vi "APD_Order.vi"(2 "APD 4":bool, 3 "APD 3":bool, 4 "APD 2":bool, 5 "APD 1":bool) -> (0 "Detectors":i32[](array[numeric]), 1 "size(s)":i32)   [LabVIEW 2010]
doc: "From combination of activated switches, outputs number of active detectors (integer) and an array with all combinations of active detectors, the values of which are set to be correctly interpreted by the FPGA."
panel:
  # "This VI outputs the number of detectors (integer) and the array\ncorresponding to all combinations of active detectors, the values\nof which are set to be correctly interpreted by the FPGA."
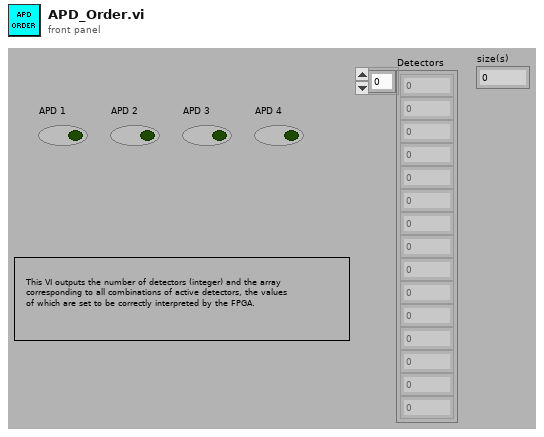
[diagram p1: front panel]
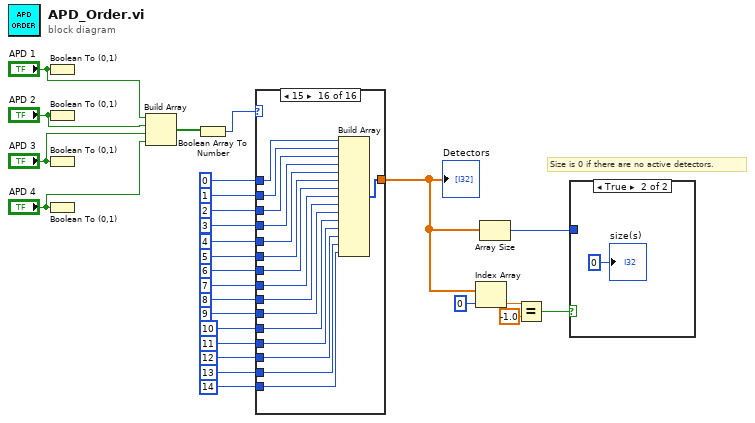
[diagram p0: block diagram]
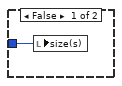
[diagram p2: hidden frame]
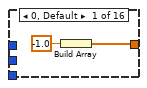
[diagram p3: hidden frame]
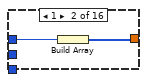
[diagram p4: hidden frame]
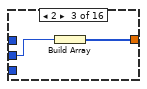
[diagram p5: hidden frame]
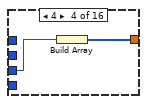
[diagram p6: hidden frame]
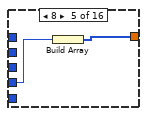
[diagram p7: hidden frame]
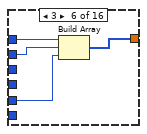
[diagram p8: hidden frame]
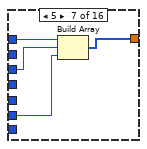
[diagram p9: hidden frame]
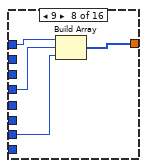
[diagram p10: hidden frame]
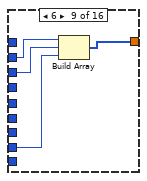
[diagram p11: hidden frame]
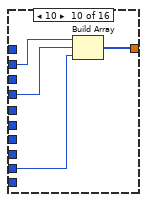
[diagram p12: hidden frame]
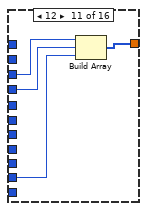
[diagram p13: hidden frame]
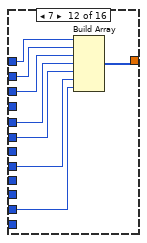
[diagram p14: hidden frame]
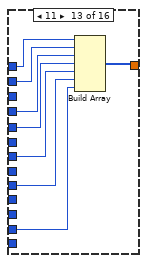
[diagram p15: hidden frame]
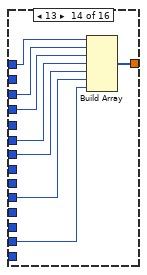
[diagram p16: hidden frame]
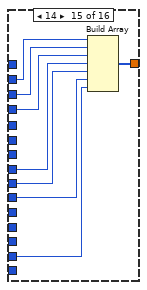
[diagram p17: hidden frame]
diagram:
  # "Size is 0 if there are no active detectors."
  n1 = Boolean To (0,1)(Boolean="APD 1") -> ()  [unwired: 1 out]
  n2 = Boolean To (0,1)(Boolean="APD 2") -> ()  [unwired: 1 out]
  n3 = Boolean To (0,1)(Boolean="APD 3") -> ()  [unwired: 1 out]
  n4 = Boolean To (0,1)(Boolean="APD 4") -> ()  [unwired: 1 out]
  n5 = Build Array("APD 1", "APD 2", "APD 3", "APD 4") -> (w26:bool[])
  n6 = Boolean Array To Number(Boolean array=w26) -> (number=w22:u32)
  n7 = case shown="15" w22 {
    tunnel: 0 -> [_ w31 _ _ _ w41 w45 w48 _ _ _ w69 w77 w85 _ w109]
    tunnel: 1 -> [_ _ w33 _ _ w40 _ _ w53 w57 _ w68 w75 _ w93 w108]
    tunnel: 2 -> [_ _ _ w35 _ _ w43 _ w52 _ w61 w67 _ w84 w92 w107]
    tunnel: 3 -> [_ _ _ _ w37 _ _ w47 _ w56 w60 _ w74 w83 w91 w106]
    tunnel: 4 -> [_ _ _ _ _ w39 _ _ _ _ _ w66 w71 _ _ w105]
    tunnel: [w28 w30 w32 w34 w36 w38 w44 w49 w50 w54 w58 w62 w70 w78 w86 w94] -> w5
    tunnel: 5 -> [_ _ _ _ _ _ w42 _ _ _ _ w65 _ w82 _ w104]
    tunnel: 6 -> [_ _ _ _ _ _ _ w46 _ _ _ _ w72 w81 _ w103]
    tunnel: 7 -> [_ _ _ _ _ _ _ _ w51 _ _ w63 _ _ w87 w102]
    tunnel: 8 -> [_ _ _ _ _ _ _ _ _ w55 _ _ w73 _ w88 w101]
    tunnel: 9 -> [_ _ _ _ _ _ _ _ _ _ w59 _ _ w80 w90 w100]
    tunnel: 10 -> [_ _ _ _ _ _ _ _ _ _ _ w64 _ _ _ w99]
    tunnel: 11 -> [_ _ _ _ _ _ _ _ _ _ _ _ w76 _ _ w98]
    tunnel: 12 -> [_ _ _ _ _ _ _ _ _ _ _ _ _ w79 _ w97]
    tunnel: 13 -> [_ _ _ _ _ _ _ _ _ _ _ _ _ _ w89 w96]
    tunnel: 14 -> [_ _ _ _ _ _ _ _ _ _ _ _ _ _ _ w95]
    frame 0, Default {
      n8 = Build Array(-1.0 ("element")) -> (w28:dbl[])
    }
    frame 1 {
      n9 = Build Array(w31) -> (w30:i32[])
    }
    frame 2 {
      n10 = Build Array(w33) -> (w32:i32[])
    }
    frame 4 {
      n11 = Build Array(w35) -> (w34:i32[])
    }
    frame 8 {
      n12 = Build Array(w37) -> (w36:i32[])
    }
    frame 3 {
      n13 = Build Array(w41, w40, w39) -> (w38:i32[])
    }
    frame 5 {
      n14 = Build Array(w45, w43, w42) -> (w44:i32[])
    }
    frame 9 {
      n15 = Build Array(w48, w47, w46) -> (w49:i32[])
    }
    frame 6 {
      n16 = Build Array(w53, w52, w51) -> (w50:i32[])
    }
    frame 10 {
      n17 = Build Array(w57, w56, w55) -> (w54:i32[])
    }
    frame 12 {
      n18 = Build Array(w61, w60, w59) -> (w58:i32[])
    }
    frame 7 {
      n19 = Build Array(w69, w68, w67, w66, w65, w63, w64) -> (w62:i32[])
    }
    frame 11 {
      n20 = Build Array(w77, w75, w74, w71, w72, w73, w76) -> (w70:i32[])
    }
    frame 13 {
      n21 = Build Array(w85, w84, w83, w82, w81, w80, w79) -> (w78:i32[])
    }
    frame 14 {
      n22 = Build Array(w93, w92, w91, w87, w88, w90, w89) -> (w86:i32[])
    }
    frame 15 {
      n23 = Build Array(w109, w108, w107, w106, w105, w104, w103, w102, w101, w100, w99, w98, w97, w96, w95) -> (w94:i32[])
    }
  }
  "Detectors" <- w5
  n24 = Index Array(array=w5, index=0) -> (element=w4:dbl)
  n25 = Array Size(array=w5) -> (size(s)=w1:i32)
  n26 = Equal?(x=w4, y=-1.0) -> (x = y?=w2:bool)
  n27 = case shown="True" w2 {
    tunnel: w1 -> [w110 _]
    frame False {
      n28 = local write "size(s)"(w110) -> ()
    }
    frame True {
      "size(s)" <- 0 ("size(s)")
    }
  }
